vi "Preprocessing.vi"() -> ()   [LabVIEW 2020]
uses:
  <vilib>/numeric/Random Number (Range) DBL.vi
panel:
  out "Potencai Ativa A 3":dbl[](array[numeric])
  out "Corrente A 3":dbl[](array[numeric])
  out "Tensão A 3":dbl[](array[numeric])
  out "Potência Ativa A 3":dbl[](graph)
  out "Potencai Ativa A 2":dbl[](array[numeric])
  out "Corrente A 2":dbl[](array[numeric])
  out "Tensão A 2":dbl[](array[numeric])
  out "Potência Ativa A 2":dbl[](graph)
  out "Potencai Ativa A":dbl[](array[numeric])
  out "Corrente A":dbl[](array[numeric])
  out "Tensão A":dbl[](array[numeric])
  out "Fator de potência":dbl
  in  "Limite inferior FP":dbl
  in  "Limite Superior FP":dbl=100.0
  out "Potência Ativa A":dbl[](graph)
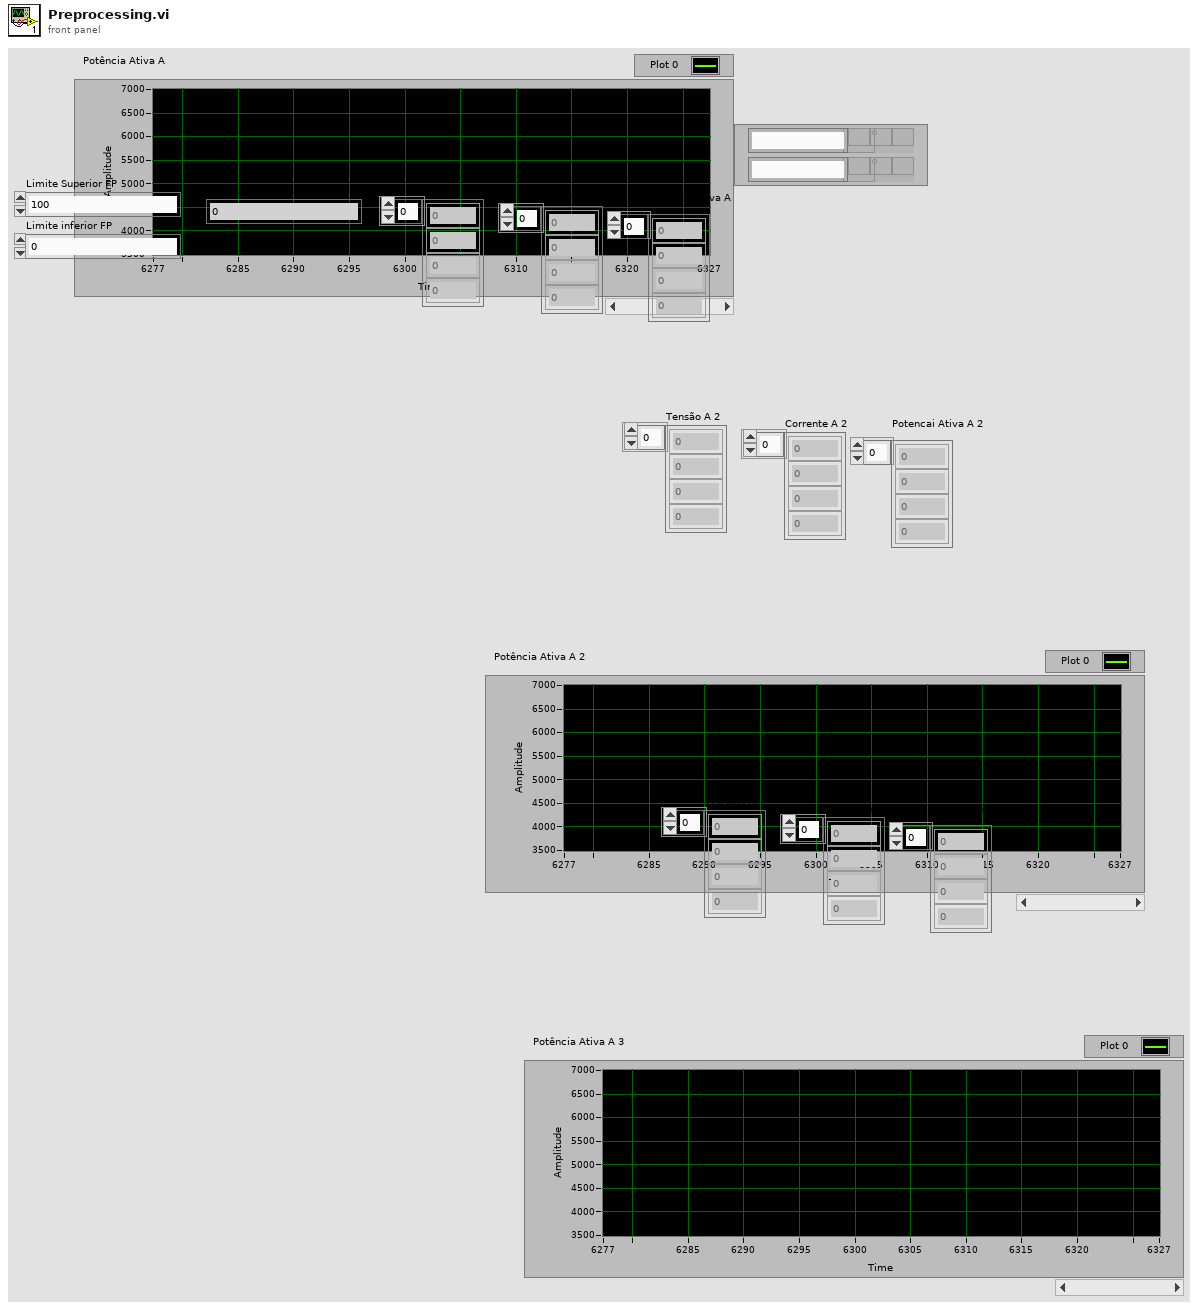
[diagram p1: front panel]
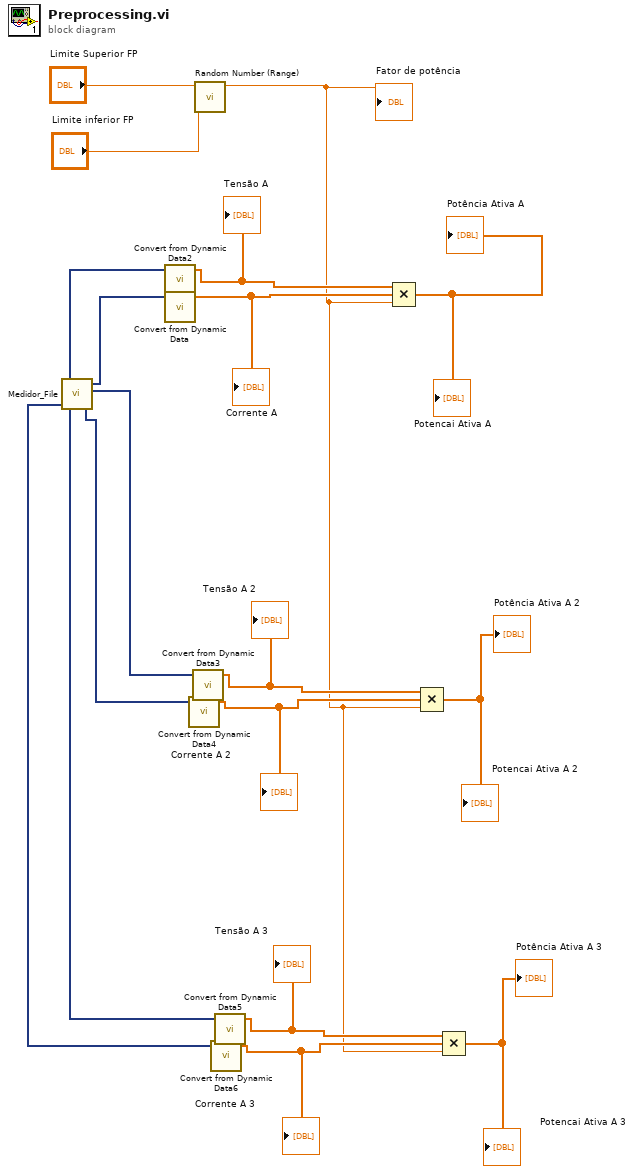
[diagram p0: block diagram]
diagram:
  n1 = call "Medidor_File.vi"() -> ("Corrente Fase C"=w2:dynamicdata, "Corrente Fase B"=w4:dynamicdata, "Corrente Fase A"=w18:dynamicdata, "Tensão Fase C"=w1:dynamicdata, "Tensão Fase B"=w3:dynamicdata, "Tensão Fase A"=w17:dynamicdata)  [unwired: 1 out]
  n2 = call "Convert from Dynamic Data2"("Dynamic Data Type"=w17) -> ("Array"=w16:dbl[])  [unwired: 3 in]
  "Tensão A" <- w16
  n3 = call "Convert from Dynamic Data"("Dynamic Data Type"=w18) -> ("Array"=w15:dbl[])  [unwired: 3 in]
  "Corrente A" <- w15
  n4 = call "Convert from Dynamic Data4"("Dynamic Data Type"=w4) -> ("Array"=w10:dbl[])  [unwired: 3 in]
  "Corrente A 2" <- w10
  n5 = call "Convert from Dynamic Data3"("Dynamic Data Type"=w3) -> ("Array"=w11:dbl[])  [unwired: 3 in]
  "Tensão A 2" <- w11
  n6 = call-poly <vilib>:"Random Number (Range).vi"("lower bound (0)"="Limite inferior FP", "upper bound (100)"="Limite Superior FP") -> ("number"=w5:dbl)  [unwired: 9 in]
  "Fator de potência" <- w5
  n7 = call "Convert from Dynamic Data6"("Dynamic Data Type"=w2) -> ("Array"=w7:dbl[])  [unwired: 3 in]
  "Corrente A 3" <- w7
  n8 = call "Convert from Dynamic Data5"("Dynamic Data Type"=w1) -> ("Array"=w8:dbl[])  [unwired: 3 in]
  "Tensão A 3" <- w8
  n9 = Compound Arithmetic op=MULTIPLY(w16, w15, w5) -> (→"Potência Ativa A" →"Potencai Ativa A":dbl[])
  n10 = Compound Arithmetic op=MULTIPLY(w11, w10, w5) -> (→"Potência Ativa A 2" →"Potencai Ativa A 2":dbl[])
  n11 = Compound Arithmetic op=MULTIPLY(w8, w7, w5) -> (→"Potência Ativa A 3" →"Potencai Ativa A 3":dbl[])
